vi "APRSClose.vi"(8 "error in (no error)":errorcluster, 11 "conRef":T1) -> (0 "error out":errorcluster)   [LabVIEW 2012]
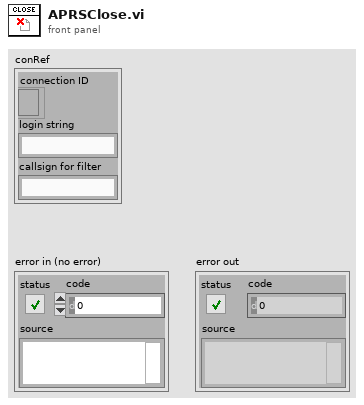
[diagram p1: front panel]
types:
  T1 = cluster{"connection ID":refnum<k5>, "login string":string, "callsign for filter":string}
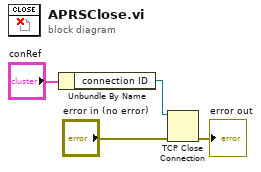
[diagram p0: block diagram]
diagram:
  n1 = Unbundle By Name("conRef") -> ("connection ID"=w1:refnum<k5>)
  n2 = TCP Close Connection(connection ID=w1, error in (no error)="error in (no error)") -> (error out=→"error out":errorcluster)  [unwired: 1 in, 1 out]
